vi "main.vi"() -> ()   [LabVIEW 2020, in "I2C Controller.lvlib"]
uses:
  I2C Controller.lvlib
  Typedef's/Main Queue Operations.ctl
  Typedef's/Main Queue State.ctl
  Classes/Common/Typedef's/Protocols Event Operations.ctl
  Typedef's/Main Data Cluster.ctl
  Classes/Parent/Protocols/Protocols.lvclass
  Classes/Parent/Protocols/Typedef's/DVR Operations.ctl
  Classes/Children/I2C/Methods/UI.vi
  Classes/Children/I2C/I2C.lvclass
panel:
  in  "Protocol":string(combo)
  in  "Error In":errorcluster
  in  "Voltage":dbl(knob)=5.0 min=0.0 max=5.0 step=0.01 scale=0.0..5.0
  in  "Frequency":dbl[unit](knob)=10000.0 min=10000.0 max=5000000.0 step=1000.0
  out "Digital Waveform":digitalwaveform(graph)
  out "Error Out":errorcluster
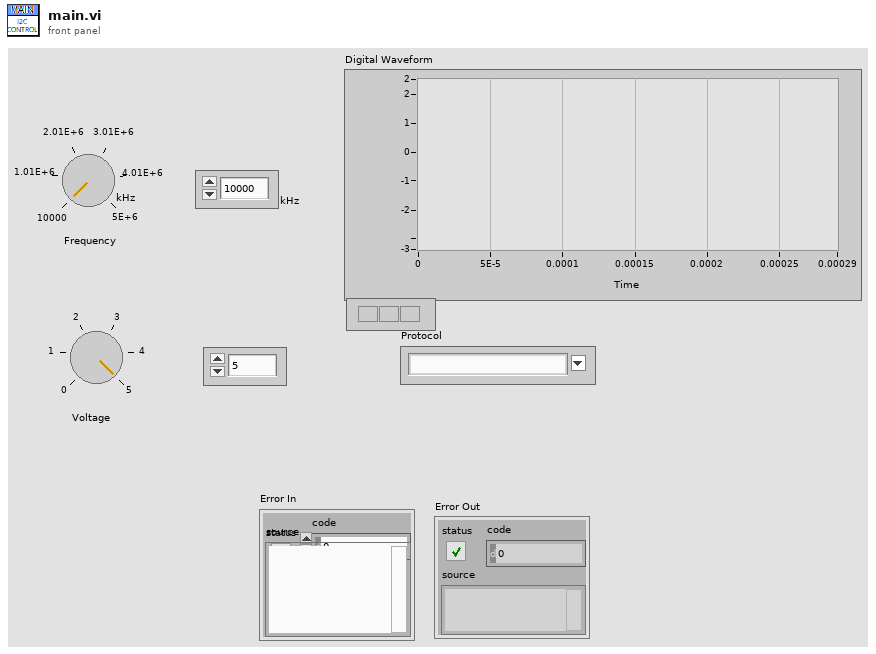
[diagram p1: front panel]
types:
  T1 = typedef "I2C Controller.lvlib/Main Data Cluster.ctl" = cluster{"Voltage":dbl, "Frequency":dbl, "Main Directory":path, "Available Protocols":string[], "Selected Protocol":string, "DVR Ref":refnum<data-value>, "Digial Waveform Data":digitalwaveform}
  T2 = typedef "I2C Controller.lvlib/Protocols Event Operations.ctl" = enum16{"Create", "Generate", "Destroy"}
  T3 = typedef "I2C Controller.lvlib/Main Queue Operations.ctl" = enum16{"Create", "Enqueue", "Dequeue", "Enstack", "Flush", "Destroy"}
  T4 = typedef "I2C Controller.lvlib/Main Queue State.ctl" = cluster{"State":string, "Data":variant}
  T5 = typedef "I2C Controller.lvlib/Protocols.lvclass/DVR Operations.ctl" = enum16{"Create", "Destroy"}
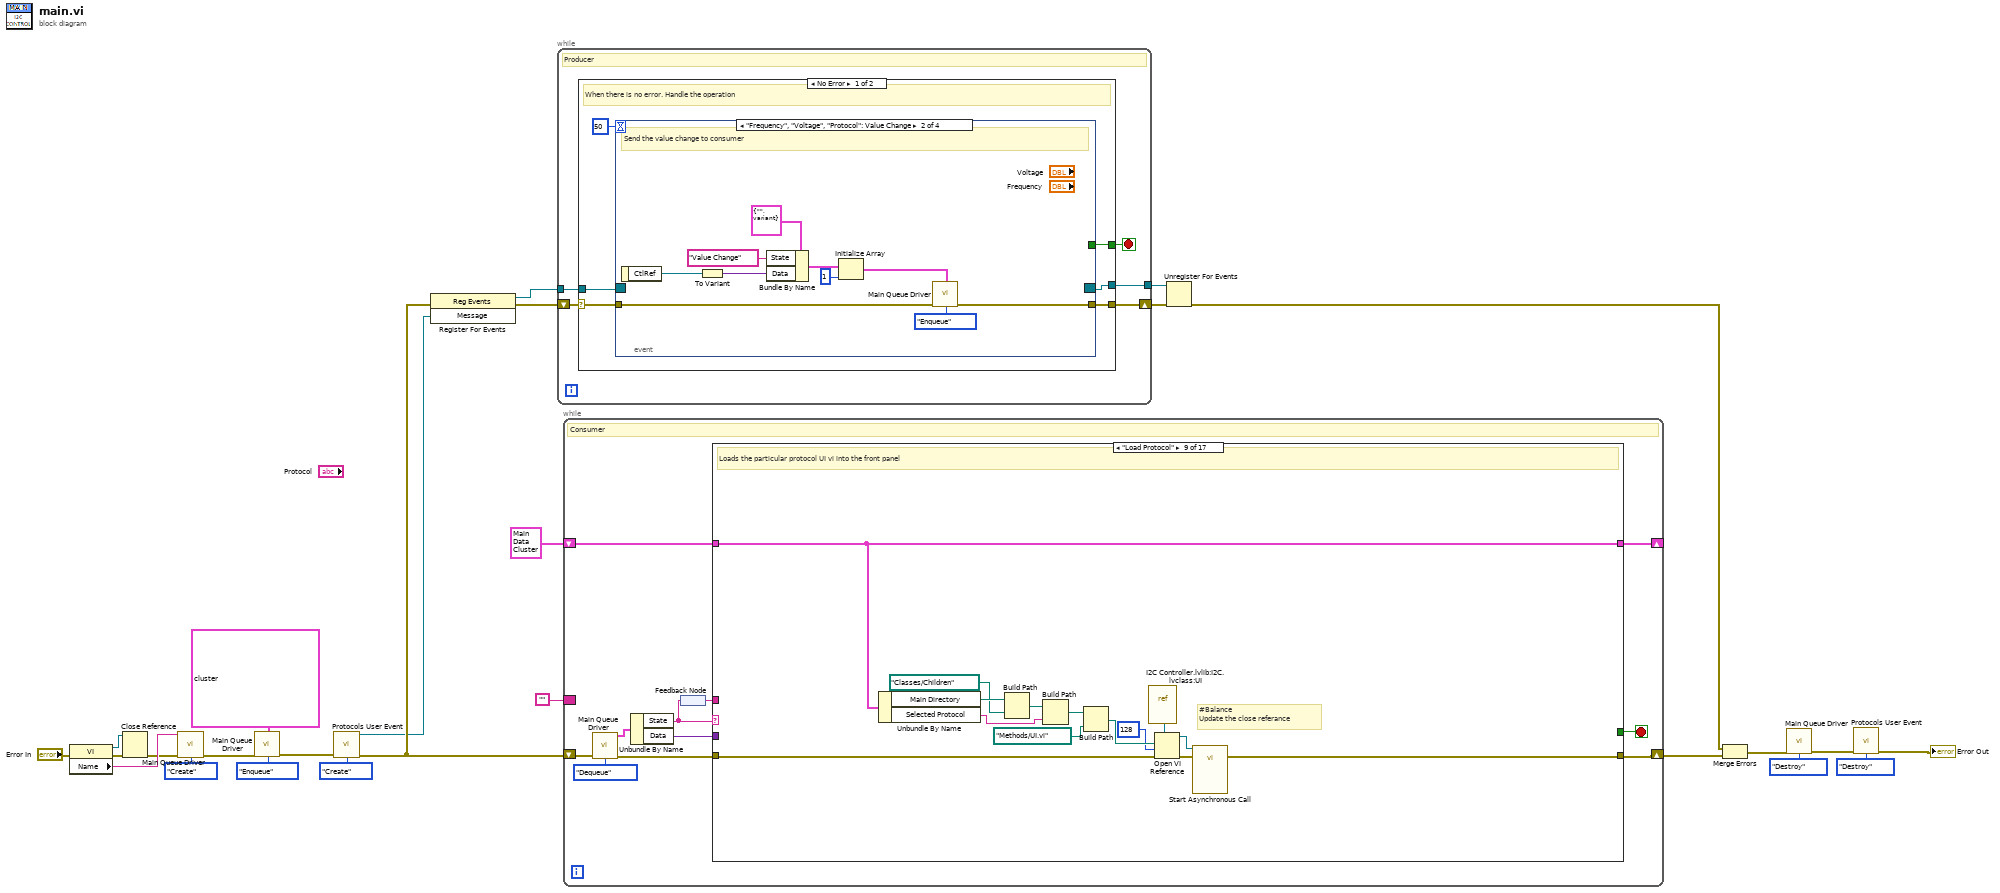
[diagram p0: block diagram]
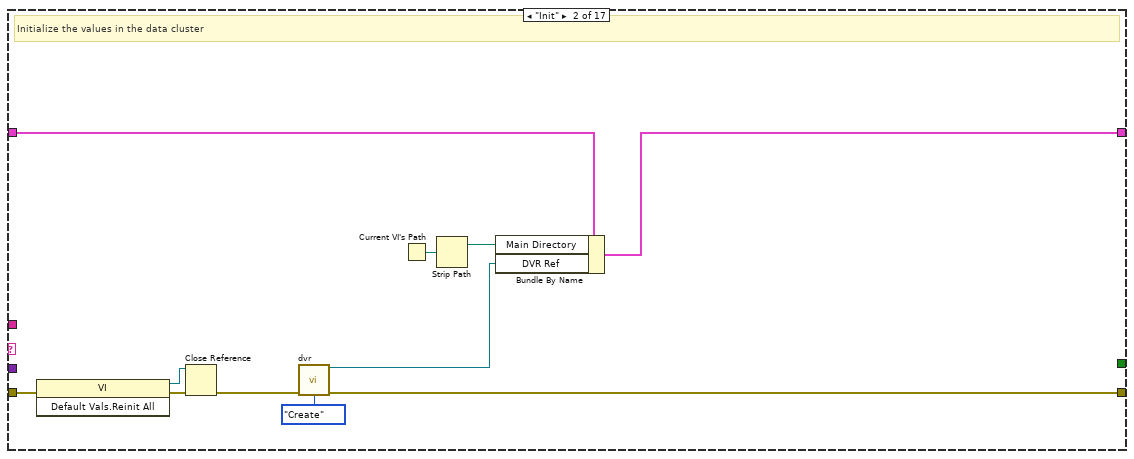
[diagram p3: hidden frame]
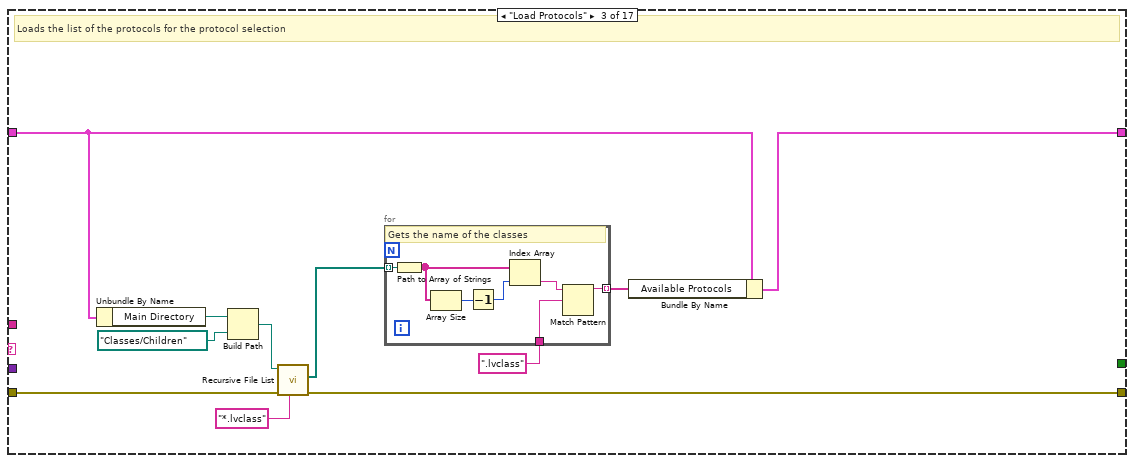
[diagram p4: hidden frame]
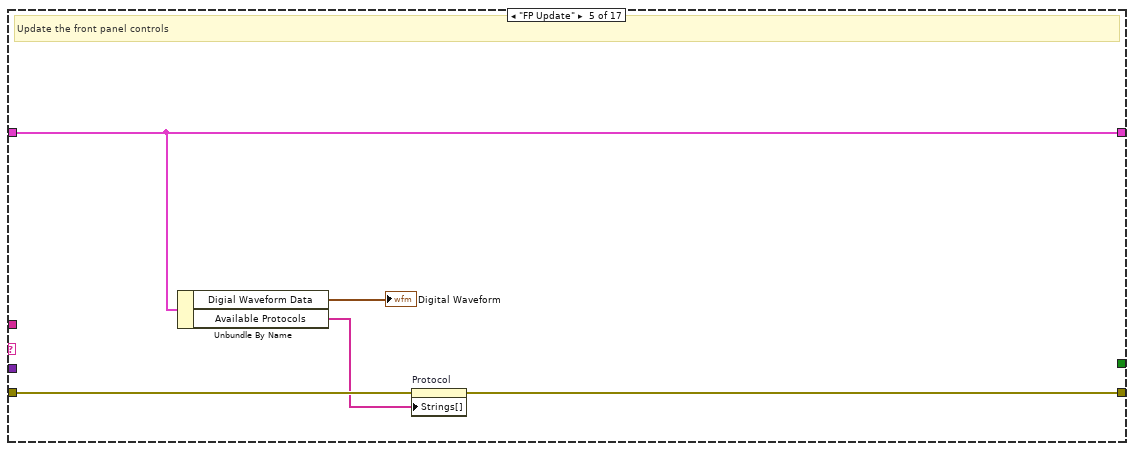
[diagram p6: hidden frame]
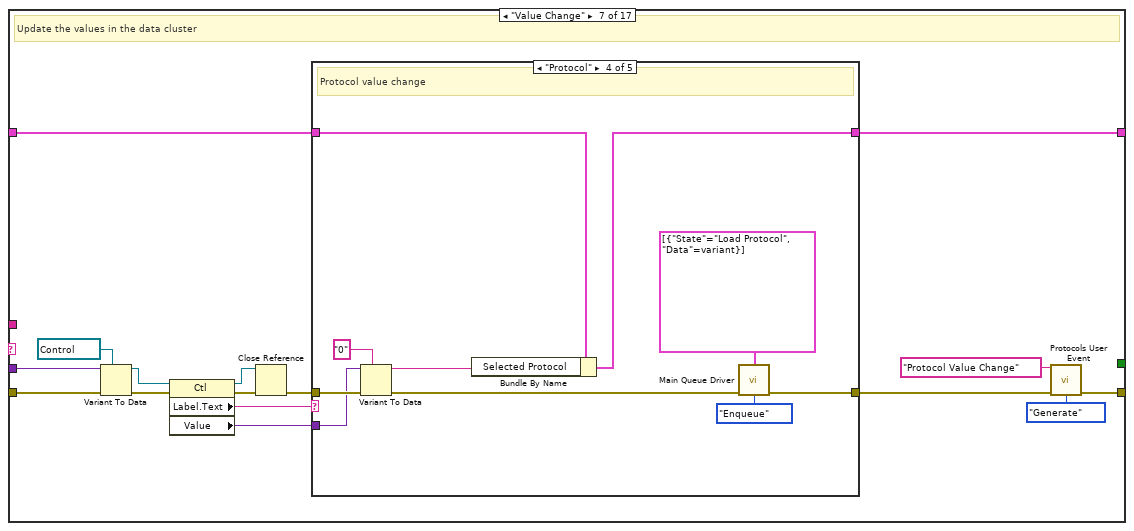
[diagram p8: hidden frame]
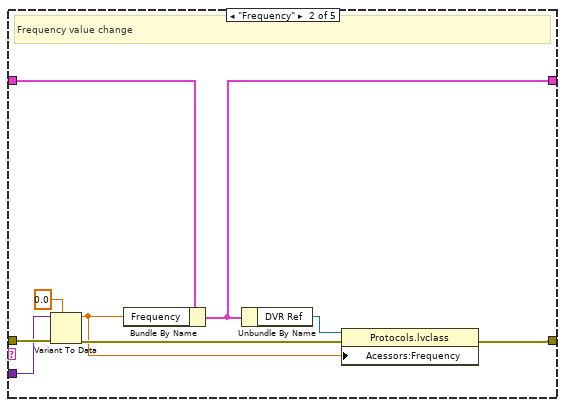
[diagram p10: hidden frame]
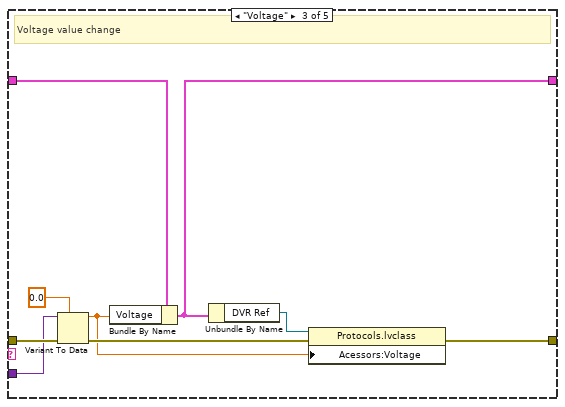
[diagram p11: hidden frame]
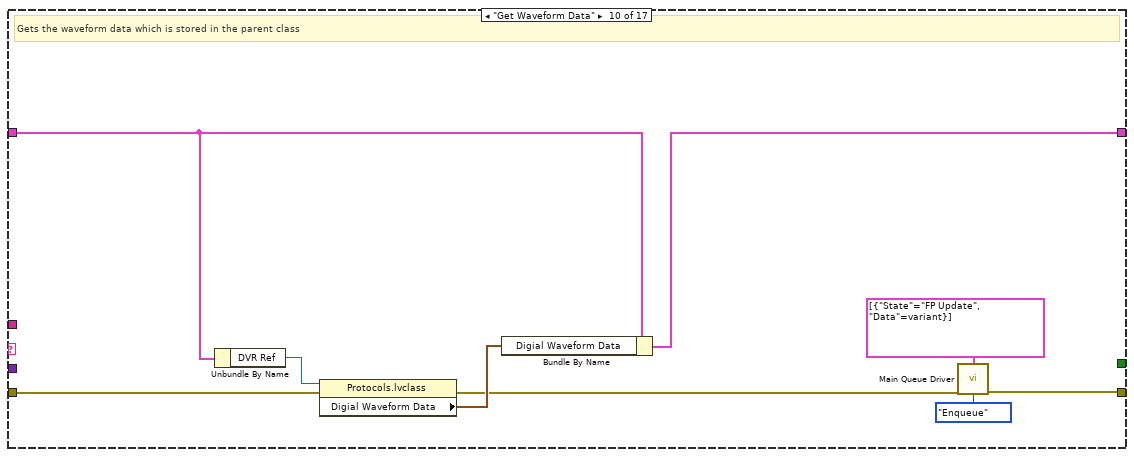
[diagram p14: hidden frame]
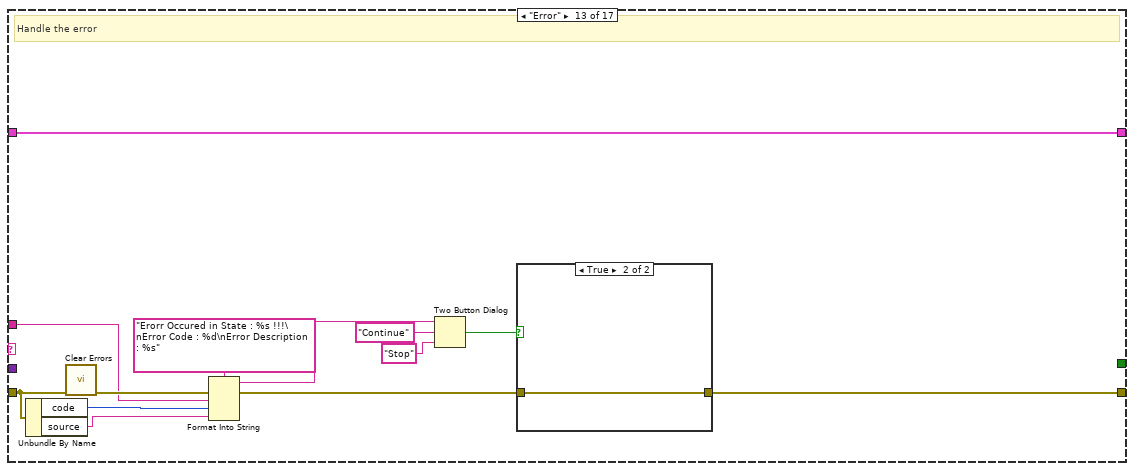
[diagram p17: hidden frame]
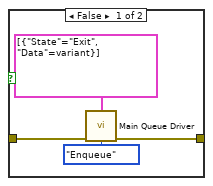
[diagram p18: hidden frame]
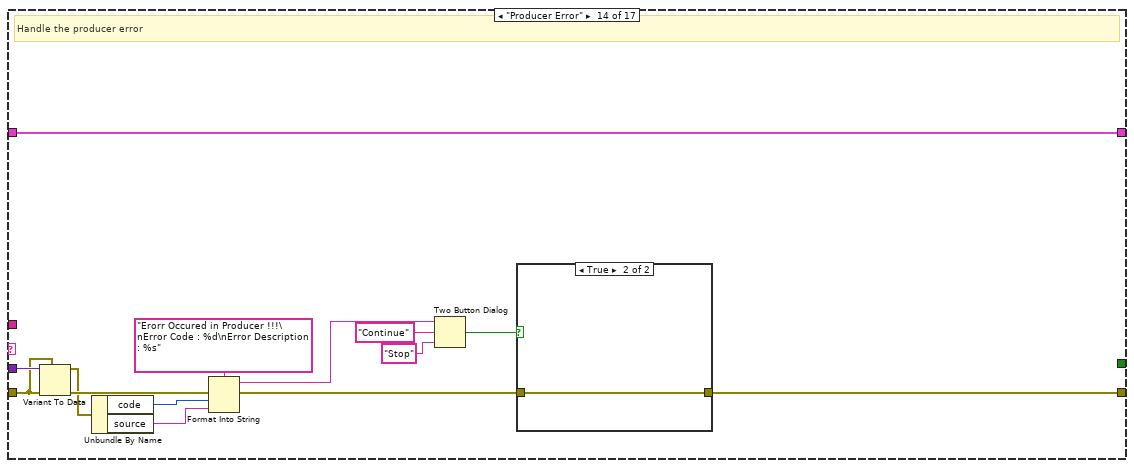
[diagram p19: hidden frame]
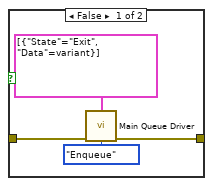
[diagram p20: hidden frame]
diagram:
  n1 = property class="VI"(error in="Error In") -> (reference out=w10:refnum<vi>, error out=w8:errorcluster, "Name"=w11:string)  [unwired: 1 in]
  n2 = Close Reference(reference=w10, error in (no error)=w8) -> (error out=w9:errorcluster)
  n3 = call "Main Queue Driver.vi"("Queue Name"=w11, "Error In"=w9, "Q Operations"=Main_Queue_Operations."Create") -> ("Error Out"=w12:errorcluster)  [unwired: 11 in, 1 out]
  n4 = call "Main Queue Driver.vi"("State[]"=T4[] [{"State"="Init", "Data"=variant}, {"State"="Load Protocols", "Data"=variant}, {"State"="FP Update", "Data"=variant}], "Error In"=w12, "Q Operations"=Main_Queue_Operations."Enqueue") -> ("Error Out"=w13:errorcluster)  [unwired: 11 in, 1 out]
  n5 = call "Protocols User Event.vi"("Error In"=w13, "Enum"=Protocols_Event_Operations."Create") -> ("Message"=w17:refnum<user-event>, "Error Out"=w18:errorcluster)  [unwired: 12 in]
  n6 = register-events(error in=w18, w17) -> (reference out=w19:refnum<event-registration>, error out=w16:errorcluster)  [unwired: 1 in]
  n7 = while {
    shift-right: [w30] -> w5
    shift-left: w16 -> [w31]
    tunnel: w19 -> [w29]
    tunnel: [w28] -> w21
    stop <- w27 stop-if-true
    # "Producer"
    n8 = case shown="No Error" w31 {
      selector: w31 -> [w37 w68]
      tunnel: [w36 w71] -> w30
      tunnel: w29 -> [w34 _]
      tunnel: [w33 _] -> w28
      tunnel: [w32 _] -> w27
      frame No Error {
        # "When there is no error. Handle the operation"
        n9 = event shown="[1] \"Frequency\", \"Voltage\", \"Protocol\": Value Change" {
          selector: w34 -> [_ _ _ _]
          dyn-events: [_ _ _ _] -> w33
          timeout: 50 -> [_ _ _ _]
          tunnel: [w38 w46 w50 w53] -> w36
          tunnel: w37 -> [w38 w47 w50 w54]
          tunnel: [_ _ _ w55] -> w32
          event Timeout {
            # "Do nothing"
            n10 = event-data() -> ()  [unwired: 1 in, 1 out]
          }
          event "Frequency", "Voltage", "Protocol": Value Change {
            # "Send the value change to consumer"
            n11 = event-data() -> ("CtlRef"=w43:refnum<vi>)  [unwired: 1 in]
            n12 = To Variant(anything=w43) -> (Variant=w42:variant)
            n13 = Bundle By Name(cluster=T4 {"State"="", "Data"=variant} ("Dequeued State"), "State"="Value Change", "Data"=w42) -> (w41:T4)
            n14 = Initialize Array(w41, 1 ("dimension size")) -> (w40:T4[])
            n15 = call "Main Queue Driver.vi"("State[]"=w40, "Error In"=w47, "Q Operations"=Main_Queue_Operations."Enqueue") -> ("Error Out"=w46:errorcluster)  [unwired: 11 in, 1 out]
          }
          event Panel Close? {
            # "Enqueue the exit operation for panel close"
            n16 = event-data() -> ()  [unwired: 1 in, 4 out]
            n17 = call "Main Queue Driver.vi"("State[]"=T4[] [{"State"="Exit", "Data"=variant}], "Error In"=w50, "Q Operations"=Main_Queue_Operations."Enqueue") -> ()  [unwired: 11 in, 2 out]
            n18 = event-data("Discard?"=TRUE) -> ()  [unwired: 1 in, 1 out]
          }
          event User Event {
            # "user generated Events"
            n19 = event-data() -> ("Message"=w56:string)  [unwired: 1 in]
            n20 = case shown="\"Update Graph\"" w56 {
              tunnel: [_ TRUE _] -> w55
              tunnel: [w57 w58 w61] -> w53
              tunnel: w54 -> [w57 w58 w62]
              frame Default {
              }
              frame "Stop All" {
              }
              frame "Update Graph" {
                n21 = call "Main Queue Driver.vi"("State[]"=T4[] [{"State"="Get Waveform Data", "Data"=variant}], "Error In"=w62, "Q Operations"=Main_Queue_Operations."Enqueue") -> ("Error Out"=w61:errorcluster)  [unwired: 11 in, 1 out]
              }
            }
          }
        }
      }
      frame Error {
        # "When there is error. Enqueue the error state"
        n22 = call <vilib>:"Clear Errors.vi"("error in (no error)"=w68) -> ("error out"=w72:errorcluster)  [unwired: 5 in, 1 out]
        n23 = To Variant(anything=w68) -> (Variant=w67:variant)
        n24 = Bundle By Name(cluster=T4 {"State"="", "Data"=variant} ("Dequeued State"), "State"="Producer Error", "Data"=w67) -> (w66:T4)
        n25 = Initialize Array(w66, 1 ("dimension size")) -> (w65:T4[])
        n26 = call "Main Queue Driver.vi"("State[]"=w65, "Error In"=w72, "Q Operations"=Main_Queue_Operations."Enqueue") -> ("Error Out"=w71:errorcluster)  [unwired: 11 in, 1 out]
      }
    }
  }
  n27 = while {
    shift-right: [w80] -> w4
    shift-left: w18 -> [w83]
    border: "" -> [_]
    shift-right: [w74] -> _
    shift-left: T1 {"Voltage"=0.0, "Frequency"=0.0, "Main Directory"=path "", "Available Protocols"=[], "Selected Protocol"="", "DVR Ref"=refnum, "Digial Waveform Data"={"t0"=timestamp(0 s since 1904-01-01), "dt"=1.0, "Y"={"transitions"=[], "data"=[]}}} -> [w75]
    stop <- w78 stop-if-true
    # "Consumer"
    n28 = call "Main Queue Driver.vi"("Error In"=w83, "Q Operations"=Main_Queue_Operations."Dequeue") -> ("Dequeued State"=w82:T4, "Error Out"=w81:errorcluster)  [unwired: 12 in]
    n29 = Unbundle By Name(w82) -> ("State"=w77:string, "Data"=w79:variant)
    n30 = feedback-in #1(w77) -> ()
    n31 = feedback #1() -> (w76:string)
    n32 = case shown="\"Load Protocol\"" w77 {
      tunnel: w81 -> [w86 w97 w108 w117 w121 w124 w140 w174 w188 w197 w199 w201 w213 w222 w242 w250 w255]
      tunnel: [w86 w89 w104 w117 w122 w124 w126 w174 w175 w190 w199 w201 w204 w226 w241 w250 w254] -> w80
      tunnel: w79 -> [_ _ _ _ _ _ w138 _ _ _ _ _ _ w223 _ _ _]
      tunnel: [_ _ _ _ _ _ _ _ _ _ _ _ _ _ _ _ TRUE] -> w78
      tunnel: w76 -> [_ _ _ _ _ _ _ _ _ _ _ _ w209 _ w243 _ _]
      tunnel: w75 -> [w85 w96 w107 w116 w120 w123 w133 w173 w187 w196 w198 w200 w202 w220 w239 w249 w251]
      tunnel: [w85 w94 w101 w116 w120 w123 w134 w173 w187 w194 w198 w200 w202 w220 w239 w249 w251] -> w74
      frame "/**** Initialization ****/" {
      }
      frame "Init" {
        # "Initialize the values in the data cluster"
        n33 = invoke class="VI" method="Default Vals.Reinit All"(error in=w97) -> (reference out=w90:refnum<vi>, error out=w92:errorcluster)  [unwired: 2 in, 1 out]
        n34 = Close Reference(reference=w90, error in (no error)=w92) -> (error out=w91:errorcluster)
        n35 = call "dvr.vi"("Error In"=w91, "DVR Operation"=DVR_Operations."Create") -> ("DVR Ref"=w87:refnum<data-value>, "Error Out"=w89:errorcluster)  [unwired: 12 in]
        n36 = Current VI's Path() -> (path=w95:path)
        n37 = Strip Path(path=w95) -> (stripped path=w93:path)  [unwired: 1 out]
        n38 = Bundle By Name(cluster=w96, "Main Directory"=w93, "DVR Ref"=w87) -> (w94:T1)
      }
      frame "Load Protocols" {
        # "Loads the list of the protocols for the protocol selection"
        n39 = Unbundle By Name(w107) -> ("Main Directory"=w106:path)
        n40 = Build Path(base path=w106, name or relative path=path "Classes/Children") -> (appended path=w103:path)
        n41 = call <vilib>:"Recursive File List.vi"("pattern"="*.lvclass", "error in (no error)"=w108, "Folder Path"=w103) -> ("error out"=w104:errorcluster, "All Files in Dir"=w102:path[])  [unwired: 4 in, 3 out]
        n42 = for {
          tunnel: w102 -> [w115] mode=indexing
          tunnel: ".lvclass" ("pattern") -> [w111]
          tunnel: [w109] -> w100 mode=indexing
          # "Gets the name of the classes"
          n43 = Path to Array of Strings(0:w115) -> (2:w114:string[])  [unwired: 1 out]
          n44 = Array Size(array=w114) -> (size(s)=w113:i32)
          n45 = Decrement(x=w113) -> (x-1=w112:i32)
          n46 = Index Array(array=w114, index=w112) -> (element=w110:string)
          n47 = Match Pattern(string=w110, regular expression=w111) -> (before substring=w109:string)  [unwired: 1 in, 3 out]
        }
        n48 = Bundle By Name(cluster=w107, "Available Protocols"=w100) -> (w101:T1)
      }
      frame "/**** FP Related *****/" {
      }
      frame "FP Update" {
        # "Update the front panel controls"
        n49 = Unbundle By Name(w120) -> ("Digial Waveform Data"=→"Digital Waveform":digitalwaveform, "Available Protocols"=w119:string[])
        n50 = property on="Protocol" class="CmbBox"(error in=w121, "Strings[]"=w119) -> (error out=w122:errorcluster)  [unwired: 1 in, 1 out]
      }
      frame "/**** Value Change ****/" {
      }
      frame "Value Change" {
        # "Update the values in the data cluster"
        n51 = Variant To Data(error in=w140, type=refnum<vi> refnum ("CtlRef"), Variant=w138) -> (data=w135:refnum<vi>, error out=w139:errorcluster)
        n52 = property class="Ctl"(reference=w135, error in=w139) -> (reference out=w129:refnum<vi>, error out=w136:errorcluster, "Label.Text"=w131:string, "Value"=w132:variant)
        n53 = Close Reference(reference=w129, error in (no error)=w136) -> (error out=w130:errorcluster)
        n54 = case shown="\"Protocol\"" w131 {
          tunnel: w130 -> [w141 w150 w160 w170 w171]
          tunnel: [w142 w143 w155 w165 w172] -> w134
          tunnel: w133 -> [w142 w151 w159 w169 w172]
          tunnel: [w141 w146 w154 w162 w171] -> w127
          tunnel: w132 -> [_ w149 w157 w168 _]
          frame "/**** Value Changes ****/" {
          }
          frame "Frequency" {
            # "Frequency value change"
            n55 = Variant To Data(error in=w150, type=0.0, Variant=w149) -> (data=w144:dbl, error out=w145:errorcluster)
            n56 = Bundle By Name(cluster=w151, "Frequency"=w144) -> (w143:T1)
            n57 = Unbundle By Name(w143) -> ("DVR Ref"=w147:refnum<data-value>)
            n58 = property class="Protocols.lvclass"(reference=w147, error in=w145, "Acessors:Frequency"=w144) -> (error out=w146:errorcluster)  [unwired: 1 out]
          }
          frame "Voltage" {
            # "Voltage value change"
            n59 = Variant To Data(error in=w160, type=0.0, Variant=w157) -> (data=w152:dbl, error out=w158:errorcluster)
            n60 = Bundle By Name(cluster=w159, "Voltage"=w152) -> (w155:T1)
            n61 = Unbundle By Name(w155) -> ("DVR Ref"=w153:refnum<data-value>)
            n62 = property class="Protocols.lvclass"(reference=w153, error in=w158, "Acessors:Voltage"=w152) -> (error out=w154:errorcluster)  [unwired: 1 out]
          }
          frame "Protocol" {
            # "Protocol value change"
            n63 = Variant To Data(error in=w170, type="0", Variant=w168) -> (data=w166:string, error out=w163:errorcluster)
            n64 = Bundle By Name(cluster=w169, "Selected Protocol"=w166) -> (w165:T1)
            n65 = call "Main Queue Driver.vi"("State[]"=T4[] [{"State"="Load Protocol", "Data"=variant}], "Error In"=w163, "Q Operations"=Main_Queue_Operations."Enqueue") -> ("Error Out"=w162:errorcluster)  [unwired: 11 in, 1 out]
          }
          frame Default {
            # "When the control name mismatches"
          }
        }
        n66 = call "Protocols User Event.vi"("Event Data"="Protocol Value Change", "Error In"=w127, "Enum"=Protocols_Event_Operations."Generate") -> ("Error Out"=w126:errorcluster)  [unwired: 11 in, 1 out]
      }
      frame "/***** functionalities ****/" {
      }
      frame "Load Protocol" {
        # "#Balance\nUpdate the close referance"
        # "Loads the particular protocol UI vi into the front panel"
        n67 = Unbundle By Name(w187) -> ("Main Directory"=w186:path, "Selected Protocol"=w183:string)
        n68 = Build Path(base path=w186, name or relative path=path "Classes/Children") -> (appended path=w184:path)
        n69 = Build Path(base path=w184, name or relative path=w183) -> (appended path=w182:path)
        n70 = Build Path(base path=w182, name or relative path=path "Methods/UI.vi") -> (appended path=w179:path)
        n71 = vi-ref "I2C Controller.lvlib:I2C.lvclass:UI.vi"() -> (w178:refnum<vi>)
        n72 = Open VI Reference(type specifier VI Refnum (for type only)=w178, vi path=w179, options=128, error in (no error)=w188) -> (vi reference=w176:refnum<vi>, error out=w180:errorcluster)  [unwired: 2 in]
        n73 = call-by-ref "Start Asynchronous Call"(reference=w176, error in=w180) -> (error out=w175:errorcluster)  [unwired: 15 in, 2 out]
      }
      frame "Get Waveform Data" {
        # "Gets the waveform data which is stored in the parent class"
        n74 = Unbundle By Name(w196) -> ("DVR Ref"=w195:refnum<data-value>)
        n75 = property class="Protocols.lvclass"(reference=w195, error in=w197) -> (error out=w189:errorcluster, "Digial Waveform Data"=w193:digitalwaveform)  [unwired: 1 out]
        n76 = Bundle By Name(cluster=w196, "Digial Waveform Data"=w193) -> (w194:T1)
        n77 = call "Main Queue Driver.vi"("State[]"=T4[] [{"State"="FP Update", "Data"=variant}], "Error In"=w189, "Q Operations"=Main_Queue_Operations."Enqueue") -> ("Error Out"=w190:errorcluster)  [unwired: 11 in, 1 out]
      }
      frame "" {
        # "Do nothing"
      }
      frame "/***** Error States ****/" {
      }
      frame "Error" {
        # "Handle the error"
        n78 = Unbundle By Name(w213) -> ("code"=w211:i32, "source"=w210:string)
        n79 = call <vilib>:"Clear Errors.vi"("error in (no error)"=w213) -> ("error out"=w214:errorcluster)  [unwired: 5 in, 1 out]
        n80 = Format Into String(format string="Erorr Occured in State : %s !!!\nError Code : %d\nError Description : %s", error in=w214, w209, w211, w210) -> (resulting string=w208:string, error out=w205:errorcluster)  [unwired: 1 in]
        n81 = Two Button Dialog(message=w208, 1:"Stop" ("F button name (\"Cancel\")"), 2:"Continue" ("T button name (\"OK\")")) -> (T button?=w203:bool)
        n82 = case shown="True" w203 {
          tunnel: w205 -> [w217 w219]
          tunnel: [w216 w219] -> w204
          frame False {
            n83 = call "Main Queue Driver.vi"("State[]"=T4[] [{"State"="Exit", "Data"=variant}], "Error In"=w217, "Q Operations"=Main_Queue_Operations."Enqueue") -> ("Error Out"=w216:errorcluster)  [unwired: 11 in, 1 out]
          }
          frame True {
          }
        }
      }
      frame "Producer Error" {
        # "Handle the producer error"
        n84 = Variant To Data(error in=w222, type=w222, Variant=w223) -> (data=w221:errorcluster, error out=w224:errorcluster)
        n85 = Unbundle By Name(w221) -> ("code"=w232:i32, "source"=w231:string)
        n86 = Format Into String(format string="Erorr Occured in Producer !!!\nError Code : %d\nError Description : %s", error in=w224, w232, w231) -> (resulting string=w230:string, error out=w227:errorcluster)  [unwired: 1 in]
        n87 = Two Button Dialog(message=w230, 1:"Stop" ("F button name (\"Cancel\")"), 2:"Continue" ("T button name (\"OK\")")) -> (T button?=w225:bool)
        n88 = case shown="True" w225 {
          tunnel: w227 -> [w236 w238]
          tunnel: [w235 w238] -> w226
          frame False {
            n89 = call "Main Queue Driver.vi"("State[]"=T4[] [{"State"="Exit", "Data"=variant}], "Error In"=w236, "Q Operations"=Main_Queue_Operations."Enqueue") -> ("Error Out"=w235:errorcluster)  [unwired: 11 in, 1 out]
          }
          frame True {
          }
        }
      }
      frame "Developer Error", Default {
        n90 = One Button Dialog(message=w243) -> (true=w240:bool)  [unwired: 1 in]
        n91 = case shown="True" w240 {
          tunnel: w242 -> [w244 w247]
          tunnel: [w244 w246] -> w241
          frame False {
          }
          frame True {
            n92 = call "Main Queue Driver.vi"("State[]"=T4[] [{"State"="Exit", "Data"=variant}], "Error In"=w247, "Q Operations"=Main_Queue_Operations."Enqueue") -> ("Error Out"=w246:errorcluster)  [unwired: 11 in, 1 out]
          }
        }
      }
      frame "/***** Exit States ****/" {
      }
      frame "Exit" {
        # "Stop all the operation and exit"
        n93 = call "Protocols User Event.vi"("Event Data"="Stop All", "Error In"=w255, "Enum"=Protocols_Event_Operations."Generate") -> ("Error Out"=w254:errorcluster)  [unwired: 11 in, 1 out]
      }
    }
  }
  n94 = Unregister For Events(event registration refnum=w21, error in=w5) -> (error out=w20:errorcluster)
  n95 = Merge Errors(w20, w4) -> (w24:errorcluster)
  n96 = call "Main Queue Driver.vi"("Error In"=w24, "Q Operations"=Main_Queue_Operations."Destroy") -> ("Error Out"=w25:errorcluster)  [unwired: 12 in, 1 out]
  n97 = call "Protocols User Event.vi"("Error In"=w25, "Enum"=Protocols_Event_Operations."Destroy") -> ("Error Out"=→"Error Out":errorcluster)  [unwired: 12 in, 1 out]
